vi "ProductUnit.vi"(5 "EndTime":timestamp, 6 "ScrappedTime":timestamp, 7 "StartTime":timestamp, 8 "error in (no error)":errorcluster, 9 "ManufacturingTime":timestamp, 10 "CreationTime":timestamp, 11 "ProductUnit in":refnum<class "ProductUnit.lvclass">) -> (0 "error out":errorcluster, 3 "Passed":bool)   [LabVIEW 2020]
uses:
  <vilib>/Averna/ProligentResultProcessor/ProligentResultProcessor.lvlibp/ProductUnit/ProductUnit.lvclass
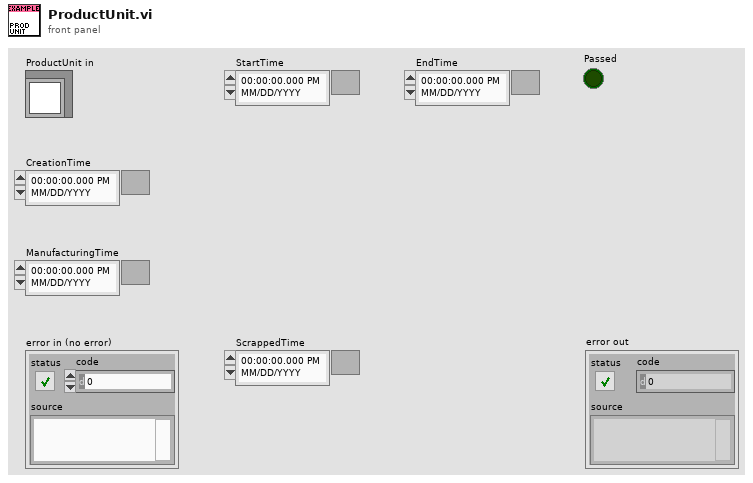
[diagram p1: front panel]
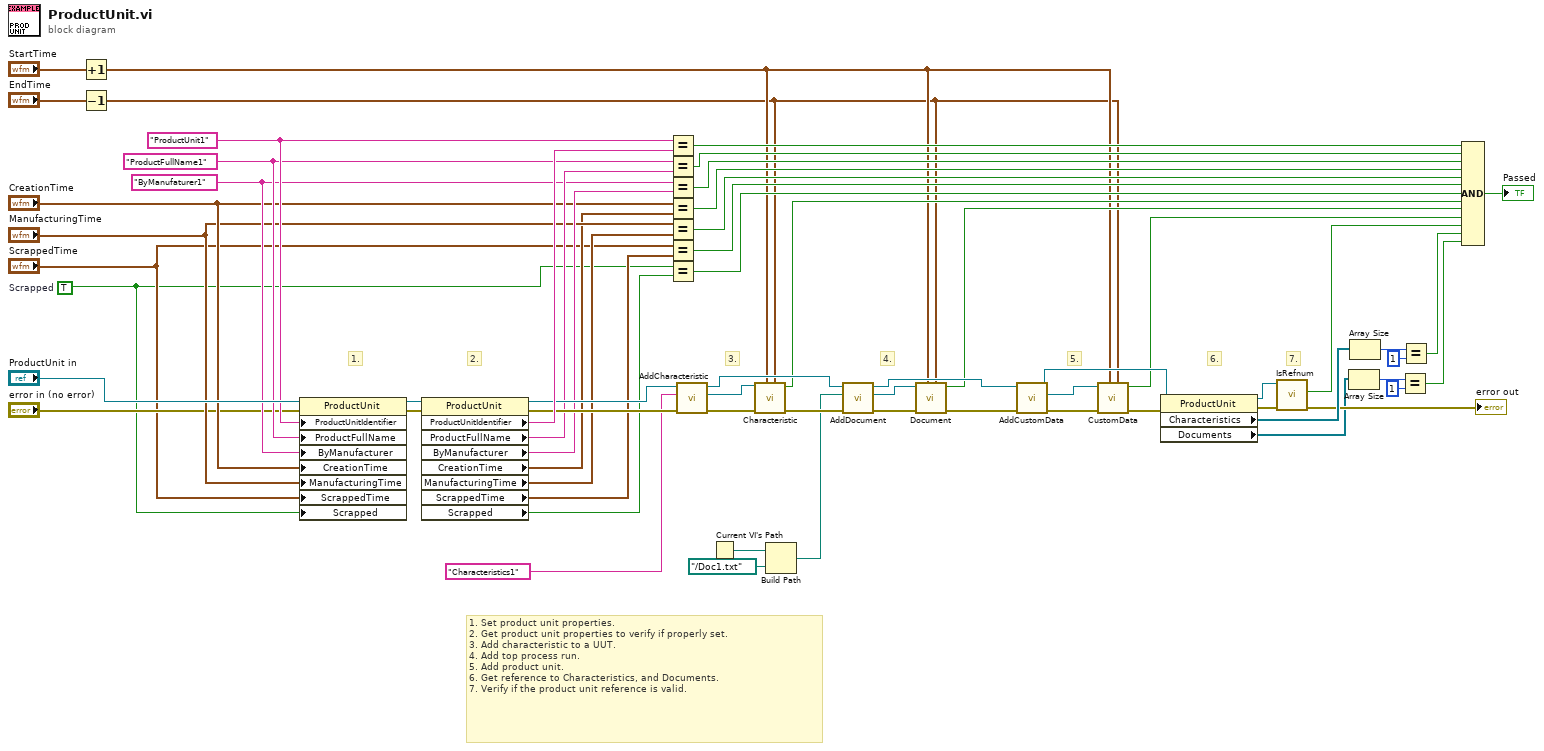
[diagram p0: block diagram]
diagram:
  w4 = TRUE  # Scrapped
  w39 = "ByManufaturer1"
  w40 = "ProductFullName1"
  w44 = "ProductUnit1"
  # "6."
  # "7."
  # "5."
  # "4."
  # "3."
  # "1. Set product unit properties.\n2. Get product unit properties to verify if properly set.\n3. Add characteristic to a UUT.\n4. Add top process run.\n5. Add product unit.\n6. Get reference to Characteristics, and Documents.\n7. Verify if the product unit reference is valid."
  # "2."
  # "1."
  n1 = Increment(x="StartTime") -> (x+1=w9:timestamp)
  n2 = Decrement(x="EndTime") -> (x-1=w8:timestamp)
  n3 = property class="ProductUnit"(reference="ProductUnit in", error in="error in (no error)", "ProductUnitIdentifier"=w44, "ProductFullName"=w40, "ByManufacturer"=w39, "CreationTime"="CreationTime", "ManufacturingTime"="ManufacturingTime", "ScrappedTime"="ScrappedTime", "Scrapped"=w4) -> (reference out=w62:refnum<class "ProductUnit.lvclass">, error out=w61:errorcluster)
  n4 = property class="ProductUnit"(reference=w62, error in=w61) -> (reference out=w50:refnum<class "ProductUnit.lvclass">, error out=w51:errorcluster, "ProductUnitIdentifier"=w59:string, "ProductFullName"=w41:string, "ByManufacturer"=w38:string, "CreationTime"=w7:timestamp, "ManufacturingTime"=w6:timestamp, "ScrappedTime"=w43:timestamp, "Scrapped"=w42:bool)
  n5 = Equal?(x=w44, y=w59) -> (x = y?=w58:bool)
  n6 = Equal?(x=w40, y=w41) -> (x = y?=w57:bool)
  n7 = Equal?(x=w39, y=w38) -> (x = y?=w56:bool)
  n8 = Equal?(x="CreationTime", y=w7) -> (x = y?=w55:bool)
  n9 = Equal?(x="ManufacturingTime", y=w6) -> (x = y?=w54:bool)
  n10 = Equal?(x="ScrappedTime", y=w43) -> (x = y?=w53:bool)
  n11 = Equal?(x=w4, y=w42) -> (x = y?=w52:bool)
  n12 = call <vilib>:"AddCharacteristic.vi"("error in"=w51, "FullName"="Characteristics1", "ProcessRun in"=w50) -> ("error out"=w16:errorcluster, "Characteristics"=w14:refnum<class "Characteristic.lvclass">, "ProcessRun out"=w17:refnum<class "ProductUnit.lvclass">)  [unwired: 6 in]
  n13 = Current VI's Path() -> (path=w3:path)
  n14 = call "Characteristic.vi"("EndTime"=w8, "StartTime"=w9, "error in (no error)"=w16, "Characteristic in"=w14) -> ("error out"=w15:errorcluster, "Passed"=w13:bool)  [unwired: 6 in]
  n15 = Build Path(base path=w3, name or relative path=path "../Doc1.txt") -> (appended path=w1:path)
  n16 = call <vilib>:"AddDocument.vi"("error in"=w15, "FilePath"=w1, "ProductUnit in"=w17) -> ("error out"=w48:errorcluster, "Characteristics"=w11:refnum<class "Document.lvclass">, "ProductUnit out"=w47:refnum<class "ProductUnit.lvclass">)  [unwired: 6 in]
  n17 = call "Document.vi"("EndTime"=w8, "StartTime"=w9, "error in (no error)"=w48, "Document in"=w11) -> ("error out"=w12:errorcluster, "Passed"=w10:bool)  [unwired: 6 in]
  n18 = call <vilib>:"AddCustomData.vi"("error in"=w12, "Defect in"=w47) -> ("error out"=w24:errorcluster, "CustomData"=w22:refnum<class "CustomData.lvclass">, "Defect out"=w45:refnum<class "ProductUnit.lvclass">)  [unwired: 7 in]
  n19 = call "CustomData.vi"("EndTime"=w8, "StartTime"=w9, "error in"=w24, "CustomData"=w22) -> ("error out"=w23:errorcluster, "Passed"=w19:bool)  [unwired: 6 in]
  n20 = property class="ProductUnit"(reference=w45, error in=w23) -> (reference out=w28:refnum<class "ProductUnit.lvclass">, error out=w35:errorcluster, "Characteristics"=w33:refnum<class "Characteristic.lvclass">[], "Documents"=w26:refnum<class "Document.lvclass">[])
  n21 = call <vilib>:"IsRefnum.vi"("error in"=w35, "ProductUnit in"=w28) -> ("error out"=→"error out":errorcluster, "IsRefnum"=w46:bool)  [unwired: 7 in, 1 out]
  n22 = Array Size(array=w26) -> (size(s)=w30:i32)
  n23 = Array Size(array=w33) -> (size(s)=w32:i32)
  n24 = Equal?(x=w30, y=1) -> (x = y?=w25:bool)
  n25 = Equal?(x=w32, y=1) -> (x = y?=w31:bool)
  n26 = Compound Arithmetic op=AND(w58, w57, w56, w55, w54, w53, w52, w13, w10, w19, w46, w31, w25) -> (→"Passed":bool)
